vi "_MainOpenMV_New.vi"() -> ()   [LabVIEW 2017]
panel:
  in  "clear":bool
  in  "Set Threshold":bool
  out "Plots":T1
  out "Lab":string="[10,90,-40,40,-40,40]"
  out "Tx Buffer":string
  in  "Play":bool
  in  "Serial Port":refnum<visa-resource-name>="ASRL30::INSTR"
  out "Version":string
  in  "Connect":bool
  out "FPS":dbl format="%#.2g"
  in  "Tabs":enum32{"Simple View", "REPL", "Python"}(tab)
  in  "WiFi":cluster{"SSID":string, "Key":string}
  in  "SystemLink":T2={"APIKey"="", "Tag"="", "Type"="STRING"}
  in  "Destination":T3(ring)
  out "Value":dbl(graph)
  in  "ROI":T4={"left"=0, "top"=0, "right"=320, "bottom"=240}
  in  "Set ROI":bool
  in  "View":T5(ring)
  in  "Ctrl D":bool
  in  "Grab Script":bool
  in  "Line":u8(slide) scale=0.0..27.0
  in  "Send Line":bool
  out "Console":string
  in  "Notepad":string
  in  "Ctrl C":bool
  out "rows":string="  1\n  2\n  3\n  4\n  5\n  6\n  7\n  8\n  9\n 10\n 11\n 12\n 13\n 14\n 15\n 16\n 17\n 18\n 19\n 20\n 21\n"
  in  "Script":string="# Show Color - lmean\n\nimport sensor, image, time\n\nsensor.reset()\nsensor.set_pixformat(sensor.RGB565)\nsensor.set_framesize(sensor.QVGA)\nsensor.skip_frames(time = 2000)\n\nsensor.set_auto_gain(False)\nsensor.set_auto_whitebal(False) \n\nclock = time.clock()\n\n\n\nwhile(True):\n    clock.tick()\n    img = sensor.snapshot()\n    \n    print(img.statistics()[0])\n"
  in  "New":bool
  in  "Load":bool
  in  "Save":bool
  in  "File":path
  in  "startCode":string="# Hello World Example\n#\n# Welcome to the OpenMV IDE! Click on the green run arrow button below to run the script!\n\nimport sensor, image, time\n\nsensor.reset()                      # Reset and initialize the sensor.\nsensor.set_pixformat(sensor.RGB565) # Set pixel format to RGB565 (or GRAYSCALE)\nsensor.set_framesize(sensor.QVGA)   # Set frame size to QVGA (320x240)\nsensor.skip_frames(time = 2000)     # Wait for settings take effect.\nclock = time.clock()                # Create a clock object to track the FPS.\n\nwhile(True):\n    clock.tick()                    # Update the FPS clock.\n    img = sensor.snapshot()         # Take a picture and return the image.\n    print(clock.fps())              # Note: OpenMV Cam runs about half as fast when connected\n                                    # to the IDE. The FPS should increase once disconnected.\n"
  out "Size":string
  in  "stop":bool
  out "image":picture
  # "LabVIEW OpenMV"
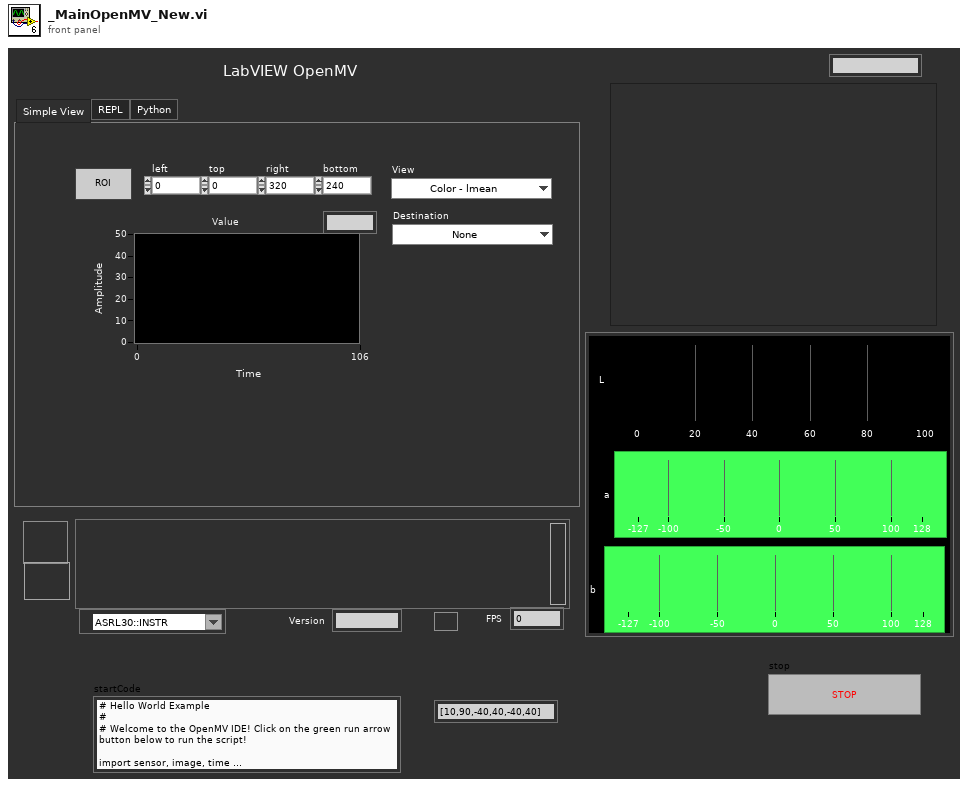
[diagram p1: front panel]
types:
  T1 = cluster{"L":dbl[], "a":cluster{i32, i32, dbl[]}, "b":cluster{i32, i32, dbl[]}}
  T2 = cluster{"APIKey":string, "Tag":string, "Type":string}
  T3 = enum16{"None", "UART (Tx-4, Rx-5)", "SPI (MOSI - 0, MISO-1, SCK-2)", "I2C (SCL-4,SDA-5)", "WiFi"}
  T4 = cluster{"left":i32, "top":i32, "right":i32, "bottom":i32}
  T5 = enum16{"Color - lmean", "Color - lmode", "Greyscale - mean", "Greyscale - mode", "Track Blobs", "Track Faces", "QRCode"}
  T6 = enum8{"Enabled", "Disabled", "Disabled and Grayed Out"}
  T7 = enum16{"Color - lmean", "Color - lmode", "Greyscale - mean", "Greyscale - mode", "Track Blobs", "Track Faces", "Optical Flow"}
  T8 = typedef "imagedata.ctl" = cluster{"image type":i32, "image depth":i32, "image":u8[], "mask":u8[], "colors":u32[], "Rectangle":cluster{"left":i16, "top":i16, "right":i16, "bottom":i16}}
  T9 = cluster{"left":i16, "top":i16, "right":i16, "bottom":i16}
  T10 = typedef "eventvkey.ctl" = enum16{"ASCII", "Enter", "Return", "Shift", "Ctrl", "Alt", "Cmd", "Opt", "Caps", "NumLock", "Clear", "Break", "Up", "Down", "Left", "Right", "Insert", "Delete", "Home", "End", "PageUp", "PageDown", "Escape", "Help", "Pause", "ScrollLock", "F1", "F2", "F3", "F4", "F5", "F6", "F7", "F8", "F9", "F10", "F11", "F12", "F13", "F14", "F15", "F16", "F17", "F18", "F19", "F20", "F21", "F22", "F23", "F24", "Play", "VolumeUp", "VolumeDown", "Mute", "Two Byte Char"}
  T11 = cluster{"Shift":bool, "Ctrl":bool, "Alt":bool, "Cmd":bool, "Opt":bool}
  T12 = cluster{"Char":i16, "VKey":T10, "ScanCode":i16, "Mods":cluster{"Num Pad":bool, "Menu Key":bool}, "PlatMods":cluster{"Shift":bool, "Ctrl":bool, "Alt":bool, "Cmd":bool, "Opt":bool}, "FocusObj":refnum<vi>}
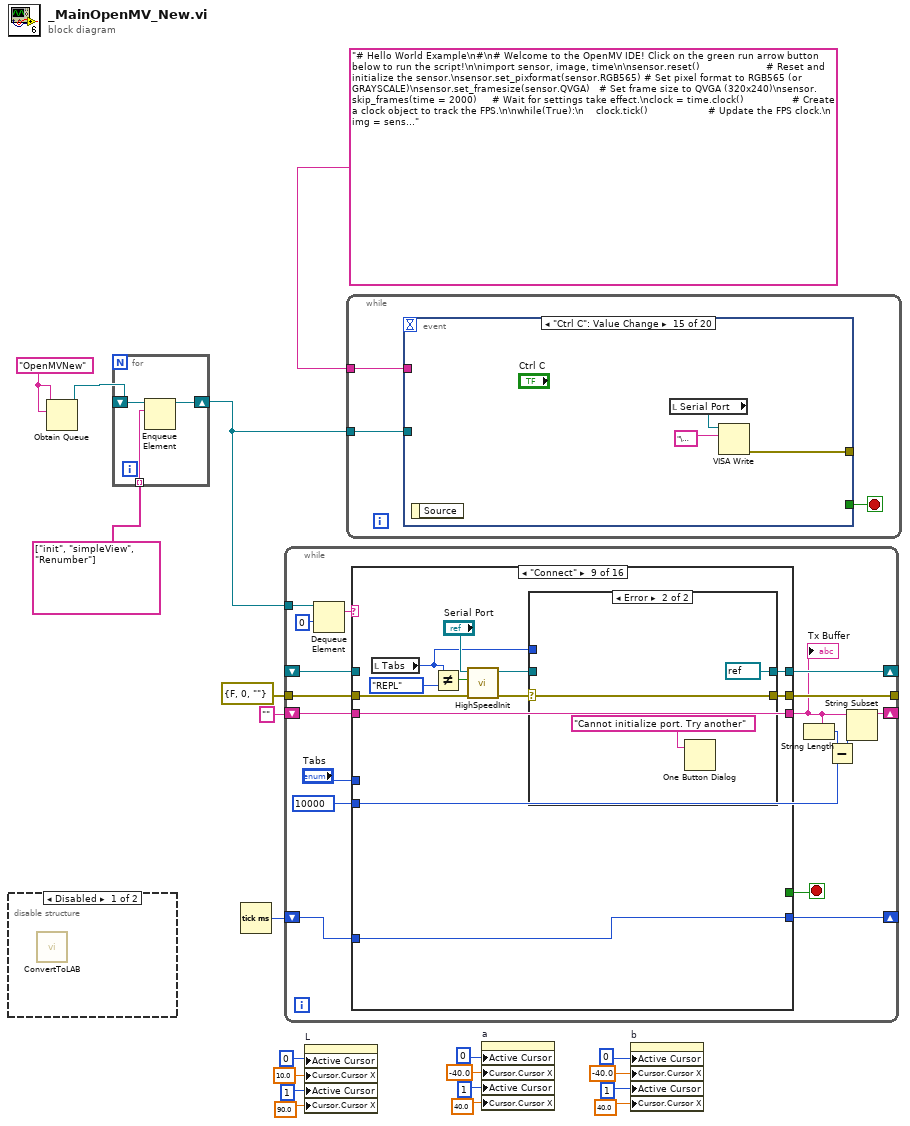
[diagram p0: block diagram]
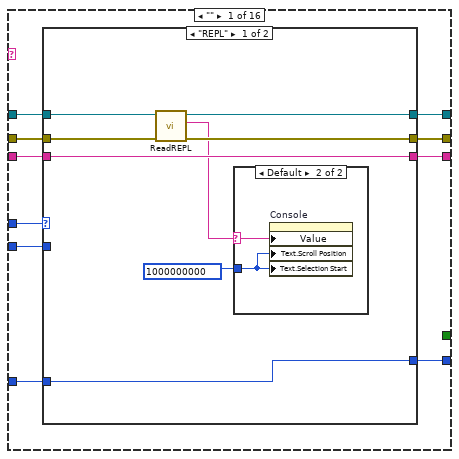
[diagram p3: hidden frame]
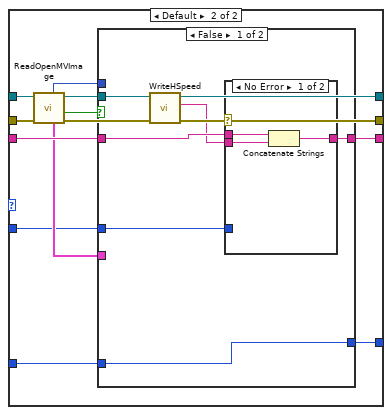
[diagram p5: hidden frame]
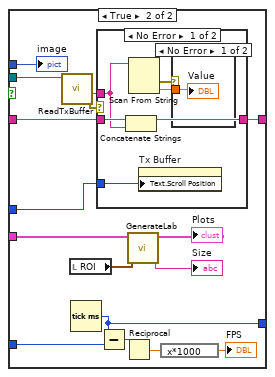
[diagram p7: hidden frame]
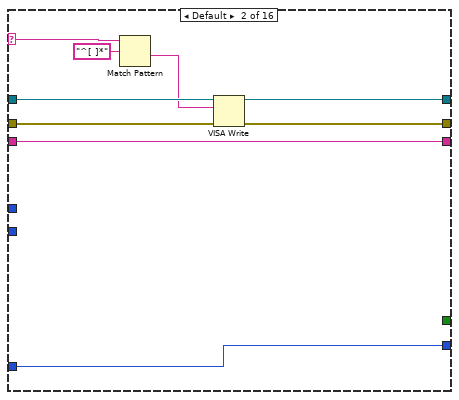
[diagram p10: hidden frame]
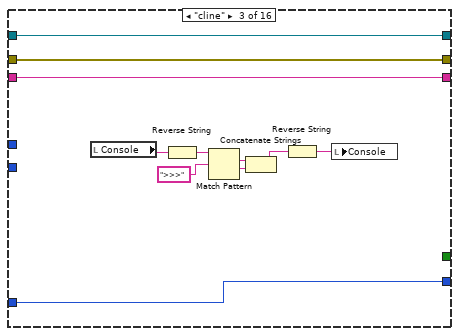
[diagram p11: hidden frame]
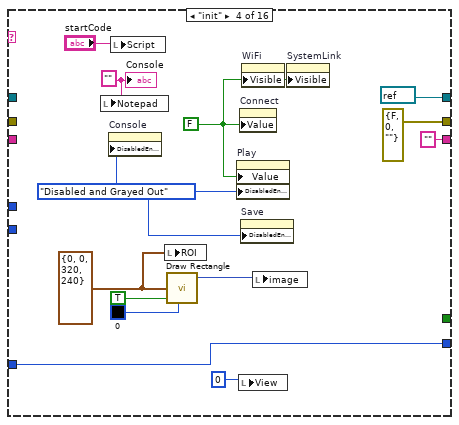
[diagram p12: hidden frame]
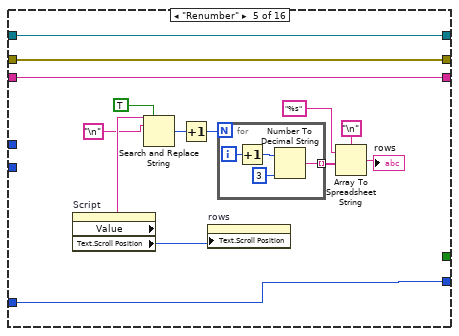
[diagram p13: hidden frame]
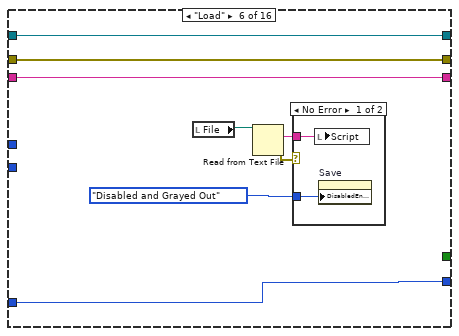
[diagram p14: hidden frame]
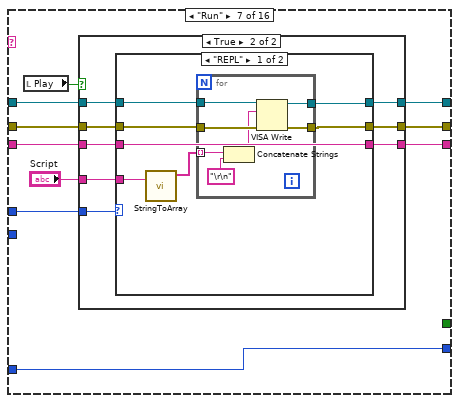
[diagram p16: hidden frame]
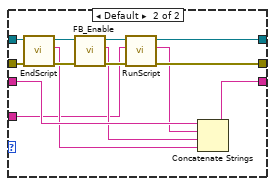
[diagram p18: hidden frame]
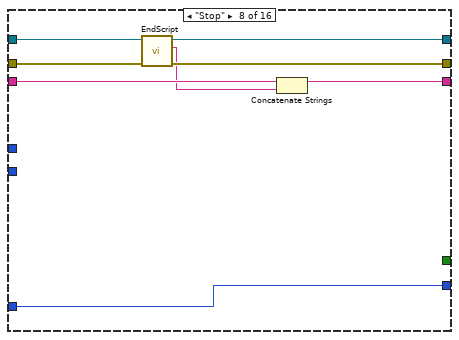
[diagram p19: hidden frame]
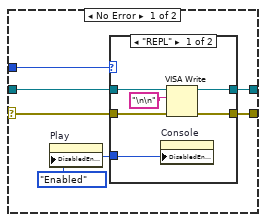
[diagram p20: hidden frame]
diagram:
  w20 = "OpenMVNew" ("name (unnamed)")
  n1 = disable-structure shown="Disabled" {
    frame Disabled {
      n2 = call <userlib>:"ConvertToLAB.vi"() -> ()  [unwired: 9 in, 3 out]
    }
    frame Enabled {
    }
  }
  n3 = Obtain Queue(name (unnamed)=w20, element data type=w20) -> (queue out=w15:refnum<queue>)  [unwired: 3 in, 2 out]
  n4 = for {
    shift-right: [w23] -> w17
    shift-left: w15 -> [w22]
    tunnel: string[] ["init", "simpleView", "Renumber"] -> [w21] mode=indexing
    n5 = Enqueue Element(queue=w22, element=w21) -> (queue out=w23:refnum<queue>)  [unwired: 2 in, 2 out]
  }
  n6 = Tick Count (ms)() -> (millisecond timer value=w18:u32)
  n7 = while {
    tunnel: w17 -> [w39]
    shift-right: [w36] -> _
    shift-left: _ -> [w37]
    shift-right: [w30] -> _
    shift-left: "" ("Tx Buffer") -> [w29]
    tunnel: errorcluster {"status"=FALSE, "code"=0, "source"=""} ("error out") -> [w34]
    tunnel: [w33] -> _
    shift-right: [w32] -> _
    shift-left: w18 -> [w31]
    stop <- w35 stop-if-true
    w27 = 10000 ("length (rest)")
    n8 = Dequeue Element(queue=w39, timeout in ms (-1)=0) -> (element=w38:string)  [unwired: 1 in, 3 out]
    n9 = case shown="\"Connect\"" w38 {
      selector: w38 -> [_ w110 _ _ _ _ _ _ _ _ _ _ _ _ _ _]
      tunnel: w37 -> [w50 w114 w125 _ w154 w166 w178 w225 _ w264 w279 w303 w311 w334 w341 w347]
      tunnel: [w47 w111 w125 refnum<visa-resource-name> refnum ("VISA Refnum out") w154 w166 w176 w222 w235 refnum<visa-resource-name> refnum ("VISA Refnum out") w279 w303 w311 w334 w341 w347] -> w36
      tunnel: [w48 w112 w124 errorcluster {"status"=FALSE, "code"=0, "source"=""} ("error out") w153 w165 w175 w223 w234 w262 w278 w302 w310 w333 w340 w346] -> w33
      tunnel: w34 -> [w49 w113 w124 _ w153 w165 w177 w224 w233 w263 w278 w302 w310 w333 w340 w346]
      tunnel: w29 -> [w46 w116 w127 _ w152 w164 w174 w219 w232 w266 w277 w301 w309 w336 _ w345]
      tunnel: [w45 w116 w127 "" ("Tx Buffer") w152 w164 w173 w220 w232 w266 w277 w301 w309 w336 "" ("Tx Buffer") w345] -> w26
      tunnel: [_ _ _ _ _ _ _ _ _ _ _ _ _ _ _ TRUE] -> w35
      tunnel: [w44 w115 w126 w137 w151 w163 w172 w221 w230 w260 w274 w300 w308 w335 w342 w343] -> w32
      tunnel: w31 -> [w43 w115 w126 w137 w151 w163 w172 w221 w230 w260 w274 w300 w308 w335 w342 w343]
      tunnel: w27 -> [w42 _ _ _ _ _ _ _ _ _ _ _ _ _ _ _]
      tunnel: "Tabs" -> [w41 _ _ _ _ _ w170 _ _ _ _ _ _ _ _ _]
      frame "" {
        n10 = case shown="\"REPL\"" w41 {
          tunnel: w50 -> [w58 w70]
          tunnel: w49 -> [w57 w69]
          tunnel: [w55 w68] -> w48
          tunnel: [w56 w67] -> w47
          tunnel: w46 -> [w54 w66]
          tunnel: [w54 w65] -> w45
          tunnel: [w53 w64] -> w44
          tunnel: w43 -> [w53 w63]
          tunnel: w42 -> [_ w61]
          frame "REPL" {
            n11 = call <userlib>:"ReadREPL.vi"("error in (no error)"=w57, "VISA Refnum in"=w58) -> ("error out"=w55:errorcluster, "String"=w51:string, "VISA Refnum out"=w56:refnum<visa-resource-name>)  [unwired: 7 in]
            n12 = case shown="Default" w51 {
              selector: w51 -> [_ w59]
              tunnel: u32 1000000000 ("Text.Selection:Start") -> [_ w60]
              frame "" {
              }
              frame Default {
                n13 = property on="Console" class="Str"("Value"=w59, "Text.Scroll Position"=w60, "Text.Selection Start"=w60) -> ()  [unwired: 2 in, 2 out]
              }
            }
          }
          frame Default {
            n14 = call <userlib>:"ReadOpenMVImage.vi"("error in"=w69, "VISA Refnum in"=w70) -> ("error out"=w68:errorcluster, "Good?"=w72:bool, "VISA Refnum out"=w67:refnum<visa-resource-name>, "image data"=w62:T8, "new picture"=w71:picture)  [unwired: 4 in, 1 out]
            n15 = case shown="False" w72 {
              tunnel: w71 -> [_ w93]
              tunnel: w67 -> [w75 w99]
              tunnel: [w77 w89] -> w65
              tunnel: w66 -> [w78 w87]
              tunnel: [w79 w98] -> w64
              tunnel: w63 -> [w79 w97]
              tunnel: w62 -> [_ w91]
              tunnel: w61 -> [w76 w84]
              frame False {
                n16 = call <userlib>:"WriteHSpeed.vi"("VISA Refnum in"=w75) -> ("error out"=w73:errorcluster, "read buffer"=w74:string)  [unwired: 8 in, 1 out]
                n17 = case shown="No Error" w73 {
                  tunnel: w74 -> [w82 _]
                  tunnel: w78 -> [w81 w83]
                  tunnel: [w80 w83] -> w77
                  tunnel: w76 -> [_ _]
                  frame No Error {
                    n18 = Concatenate Strings(w81, w82) -> (w80:string)
                  }
                  frame Error {
                  }
                }
              }
              frame True {
                n19 = call <userlib>:"ReadTxBuffer.vi"("VISA Refnum in"=w99) -> ("error out"=w85:errorcluster, "Tx Buffer"=w86:string)  [unwired: 7 in, 2 out]
                n20 = local read "ROI"() -> (w90:T4)
                n21 = Tick Count (ms)() -> (millisecond timer value=w98:u32)
                n22 = case shown="No Error" w85 {
                  tunnel: [w105 w107] -> w89
                  tunnel: w87 -> [w102 w107]
                  tunnel: w86 -> [w101 _]
                  tunnel: w84 -> [w100 _]
                  frame No Error {
                    n23 = Concatenate Strings(w102, w101) -> (w105:string)
                    n24 = Scan From String(input string=w101) -> (error out=w104:errorcluster, output 1=w103:dbl)  [unwired: 4 in, 2 out]
                    n25 = property on="Tx Buffer" class="Str"("Text.Scroll Position"=w100) -> ()  [unwired: 2 in, 2 out]
                    n26 = case shown="No Error" w104 {
                      tunnel: w103 -> [w106 _]
                      frame No Error {
                        "Value" <- w106
                      }
                      frame Error {
                      }
                    }
                  }
                  frame Error {
                  }
                }
                n27 = Subtract(x=w98, y=w97) -> (x-y=w94:u32)
                n28 = Reciprocal(x=w94) -> (1/x=w96:dbl)
                n29 = call <userlib>:"GenerateLab.vi"("ROI"=w90, "image data"=w91) -> ("Dimensions"=→"Size":string, "Plots"=→"Plots":T1)  [unwired: 8 in]
                n30 = expression code="x*1000"(w96) -> (→"FPS":dbl)
                "image" <- w93
              }
            }
          }
        }
      }
      frame Default {
        n31 = Match Pattern(string=w110, regular expression="^[ ]*") -> (after substring=w109:string)  [unwired: 1 in, 3 out]
        n32 = VISA Write(VISA resource name=w114, write buffer=w109, error in (no error)=w113) -> (VISA resource name out=w111:refnum<visa-resource-name>, error out=w112:errorcluster)  [unwired: 1 out]
      }
      frame "cline" {
        n33 = local read "Console"() -> (w117:string)
        n34 = Reverse String(1:w117) -> (0:w123:string)
        n35 = Match Pattern(string=w123, regular expression=">>>") -> (match substring=w120:string, after substring=w121:string)  [unwired: 1 in, 2 out]
        n36 = Concatenate Strings(w120, w121) -> (w119:string)
        n37 = Reverse String(1:w119) -> (0:w118:string)
        n38 = local write "Console"(w118) -> ()
      }
      frame "init" {
        w130 = "" ("Tx Buffer")
        w132 = T9 {"left"=0, "top"=0, "right"=320, "bottom"=240} ("rect")
        w129 = T6."Disabled and Grayed Out" ("Disabled")
        w131 = FALSE ("Connect")
        n39 = local write "Notepad"(w130) -> ()
        n40 = property on="Console" class="Str"("DisabledEnum"=w129) -> ()  [unwired: 2 in, 2 out]
        n41 = local write "Script"("startCode") -> ()
        n42 = local write "ROI"(w132) -> ()
        n43 = call <vilib>:"Draw Rectangle.vi"("rect"=w132, "fill?(F)"=TRUE, "color(black)"=u32 0) -> ("new picture"=w134:picture)  [unwired: 6 in]
        n44 = property on="Play" class="Bool (strict)"("Value"=w131, "DisabledEnum"=w129) -> ()  [unwired: 2 in, 2 out]
        n45 = local write "View"(i16 0 ("left")) -> ()
        n46 = property on="Connect" class="Bool (strict)"("Value"=w131) -> ()  [unwired: 2 in, 2 out]
        n47 = property on="Save" class="Bool"("DisabledEnum"=w129) -> ()  [unwired: 2 in, 2 out]
        n48 = property on="WiFi" class="Clust (strict)"("Visible"=w131) -> ()  [unwired: 2 in, 2 out]
        n49 = local write "image"(w134) -> ()
        n50 = property on="SystemLink" class="Clust (strict)"("Visible"=w131) -> ()  [unwired: 2 in, 2 out]
        "Console" <- w130
      }
      frame "Renumber" {
        n51 = property on="Script" class="Str"() -> ("Value"=w150:string, "Text.Scroll Position"=w149:u32)  [unwired: 2 in, 2 out]
        n52 = Search and Replace String(replace all?=TRUE ("replace all? (F)"), input string=w150, search string="\n") -> (number of replacements=w148:i32)  [unwired: 5 in, 3 out]
        n53 = Increment(x=w148) -> (x+1=w141:i32)
        n54 = property on="rows" class="Str"("Text.Scroll Position"=w149) -> ()  [unwired: 2 in, 2 out]
        n55 = for {
          N: w141 -> [_]
          tunnel: [w158] -> w146 mode=indexing
          i -> [w155]
          n56 = Increment(x=w155) -> (x+1=w157:i32)
          n57 = Number To Decimal String(number=w157, width (-)=i16 3) -> (decimal integer string=w158:string)
        }
        n58 = Array To Spreadsheet String(delimiter (Tab)="\n", array=w146, 3:"%s" ("format string")) -> (spreadsheet string=→"rows":string)
      }
      frame "Load" {
        n59 = local read "File"() -> (w162:path)
        n60 = Read from Text File(file (use dialog)=w162) -> (text=w159:string, error out=w160:errorcluster)  [unwired: 3 in, 2 out]
        n61 = case shown="No Error" w160 {
          tunnel: T6."Disabled and Grayed Out" ("Disabled") -> [w168 _]
          tunnel: w159 -> [w167 _]
          frame No Error {
            n62 = local write "Script"(w167) -> ()
            n63 = property on="Save" class="Bool"("DisabledEnum"=w168) -> ()  [unwired: 2 in, 2 out]
          }
          frame Error {
          }
        }
      }
      frame "Run" {
        n64 = local read "Play"() -> (w171:bool)
        n65 = case shown="True" w171 {
          tunnel: w178 -> [w181 w189]
          tunnel: w177 -> [w180 w188]
          tunnel: [w181 w187] -> w176
          tunnel: [w180 w186] -> w175
          tunnel: w174 -> [w179 w184]
          tunnel: [w179 w185] -> w173
          tunnel: w170 -> [_ w183]
          tunnel: "Script" -> [_ w182]
          frame False {
          }
          frame True {
            n66 = case shown="\"REPL\"" w183 {
              tunnel: w189 -> [w195 w213]
              tunnel: w188 -> [w194 w212]
              tunnel: [w192 w211] -> w187
              tunnel: [w193 w210] -> w186
              tunnel: [w190 w209] -> w185
              tunnel: w184 -> [w190 w208]
              tunnel: w182 -> [w191 w204]
              frame "REPL" {
                n67 = call <userlib>:"StringToArray.vi"("write buffer"=w191) -> ("Array"=w196:string[])  [unwired: 10 in]
                n68 = for {
                  tunnel: w196 -> [w198] mode=indexing
                  tunnel: w195 -> [w203]
                  tunnel: w194 -> [w202]
                  tunnel: [w201] -> w193
                  tunnel: [w200] -> w192
                  n69 = Concatenate Strings(w198, "\r\n" ("write buffer")) -> (w197:string)
                  n70 = VISA Write(VISA resource name=w203, write buffer=w197, error in (no error)=w202) -> (VISA resource name out=w200:refnum<visa-resource-name>, error out=w201:errorcluster)  [unwired: 1 out]
                }
              }
              frame Default {
                n71 = call <userlib>:"EndScript.vi"("error in (no error)"=w212, "VISA Refnum in"=w213) -> ("error out"=w217:errorcluster, "Tx for stopping code"=w205:string, "VISA Refnum out"=w216:refnum<visa-resource-name>)  [unwired: 7 in]
                n72 = call <userlib>:"FB_Enable.vi"("error in"=w217, "VISA Refnum in"=w216) -> ("error out"=w215:errorcluster, "Reply"=w206:string, "VISA Refnum out"=w214:refnum<visa-resource-name>)  [unwired: 7 in]
                n73 = call <userlib>:"RunScript.vi"("error in"=w215, "script"=w204, "VISA Refnum in"=w214) -> ("error out"=w210:errorcluster, "Tx"=w207:string, "VISA Refnum out"=w211:refnum<visa-resource-name>)  [unwired: 6 in]
                n74 = Concatenate Strings(w208, w207, w206, w205) -> (w209:string)
              }
            }
          }
        }
      }
      frame "Stop" {
        n75 = call <userlib>:"EndScript.vi"("error in (no error)"=w224, "VISA Refnum in"=w225) -> ("error out"=w223:errorcluster, "Tx for stopping code"=w218:string, "VISA Refnum out"=w222:refnum<visa-resource-name>)  [unwired: 7 in]
        n76 = Concatenate Strings(w219, w218) -> (w220:string)
      }
      frame "Connect" {
        n77 = local read "Tabs"() -> (w227:enum32{"Simple View", "REPL", "Python"})
        n78 = Not Equal?(x=w227, y=enum32{"Simple View", "REPL", "Python"}."REPL") -> (x != y?=w229:bool)
        n79 = call <userlib>:"HighSpeedInit.vi"("error in"=w233, "Fast"=w229, "VISA Refnum in"="Serial Port") -> ("error out"=w226:errorcluster, "VISA Refnum out"=w236:refnum<visa-resource-name>)  [unwired: 7 in]
        n80 = case shown="Error" w226 {
          selector: w226 -> [w237 w255]
          tunnel: w236 -> [w242 _]
          tunnel: [w241 refnum<visa-resource-name> refnum ("VISA Refnum out")] -> w235
          tunnel: [w240 w255] -> w234
          tunnel: w227 -> [w239 _]
          frame No Error {
            w238 = T6."Enabled" ("Disabled")
            n81 = property on="Play" class="Bool (strict)"("DisabledEnum"=w238) -> ()  [unwired: 2 in, 2 out]
            n82 = case shown="\"REPL\"" w239 {
              tunnel: w237 -> [w246 w253]
              tunnel: w242 -> [w248 w252]
              tunnel: [w244 w250] -> w241
              tunnel: [w245 w249] -> w240
              tunnel: w238 -> [w243 _]
              frame "REPL" {
                n83 = property on="Console" class="Str"("DisabledEnum"=w243) -> ()  [unwired: 2 in, 2 out]
                n84 = VISA Write(VISA resource name=w248, write buffer="\n\n", error in (no error)=w246) -> (VISA resource name out=w244:refnum<visa-resource-name>, error out=w245:errorcluster)  [unwired: 1 out]
              }
              frame Default {
                n85 = call <userlib>:"AskVersion.vi"("error in"=w253, "VISA Refnum in"=w252) -> ("error out"=w249:errorcluster, "Version"=→"Version":string, "VISA Refnum out"=w250:refnum<visa-resource-name>)  [unwired: 7 in]
              }
            }
          }
          frame Error {
            n86 = One Button Dialog(message="Cannot initialize port. Try another") -> ()  [unwired: 1 in, 1 out]
          }
        }
      }
      frame "Disconnect" {
        w257 = T6."Disabled and Grayed Out" ("Disabled")
        n87 = local read "Tabs"() -> (w258:enum32{"Simple View", "REPL", "Python"})
        n88 = case shown="\"REPL\"" w258 {
          tunnel: [w269 w273] -> w265
          tunnel: w264 -> [w269 w272]
          tunnel: w263 -> [w268 w271]
          tunnel: [w268 w270] -> w262
          frame "REPL" {
          }
          frame Default {
            n89 = call <userlib>:"EndScript.vi"("error in (no error)"=w271, "VISA Refnum in"=w272) -> ("error out"=w270:errorcluster, "VISA Refnum out"=w273:refnum<visa-resource-name>)  [unwired: 7 in, 1 out]
          }
        }
        n90 = call <userlib>:"CloseHS.vi"("error in (no error)"=w262, "VISA Refnum in"=w265) -> ()  [unwired: 10 in]
        n91 = local write "Connect"(FALSE ("Connect")) -> ()
        n92 = property on="Play" class="Bool (strict)"("Value"=FALSE ("Play"), "DisabledEnum"=w257) -> ()  [unwired: 2 in, 2 out]
        n93 = property on="Console" class="Str"("DisabledEnum"=w257) -> ()  [unwired: 2 in, 2 out]
      }
      frame "ROI" {
        n94 = local read "image"() -> (w275:picture)
        n95 = call <userlib>:"OpenMV_SelectROI.vi"("image"=w275) -> ("Rect"=w276:T4)  [unwired: 2 in]
        n96 = local write "ROI"(w276) -> ()
      }
      frame "Lab" {
        n97 = property on="L" class="WFGraph (strict)"("Active Cursor"=u32 0, "Active Cursor"=u32 1) -> ("Cursor.Cursor X"=w293:dbl, "Cursor.Cursor X"=w292:dbl)  [unwired: 2 in, 2 out]
        n98 = property on="a" class="WFGraph (strict)"("Active Cursor"=u32 0, "Active Cursor"=u32 1) -> ("Cursor.Cursor X"=w294:dbl, "Cursor.Cursor X"=w295:dbl)  [unwired: 2 in, 2 out]
        n99 = property on="b" class="WFGraph (strict)"("Active Cursor"=u32 0, "Active Cursor"=u32 1) -> ("Cursor.Cursor X"=w296:dbl, "Cursor.Cursor X"=w297:dbl)  [unwired: 2 in, 2 out]
        n100 = Max & Min(x=w293, y=w292) -> (max(x,y)=w285:dbl, min(x,y)=w284:dbl)
        n101 = Max & Min(x=w294, y=w295) -> (max(x,y)=w283:dbl, min(x,y)=w282:dbl)
        n102 = Max & Min(x=w296, y=w297) -> (max(x,y)=w280:dbl, min(x,y)=w281:dbl)
        n103 = Format Into String(format string="[%d,%d,%d,%d,%d,%d]", w284, w285, w282, w283, w281, w280) -> (resulting string=→"Lab":string)  [unwired: 2 in, 1 out]
      }
      frame "LabPopup" {
        n104 = local read "image"() -> (w306:picture)
        n105 = local read "ROI"() -> (w304:T4)
        n106 = call <userlib>:"OpenMV_SelectLab.vi"("ROI"=w304, "image"=w306) -> ("ROI out"=w305:T4, "thresholds"=w307:dbl[])
        n107 = for {
          tunnel: w307 -> [w312] mode=indexing
          i -> [w316]
          n108 = Quotient & Remainder(x=w316, y=2) -> (x-y*floor(x/y)=w313:i32, floor(x/y)=w314:i32)
          n109 = case shown="0" w314 {
            tunnel: w313 -> [_ w318 w320 w322]
            tunnel: w312 -> [_ w317 w319 w321]
            frame Default {
            }
            frame 0 {
              n110 = property on="L" class="WFGraph (strict)"("Active Cursor"=w318, "Cursor.Cursor X"=w317) -> ()  [unwired: 2 in, 2 out]
            }
            frame 1 {
              n111 = property on="a" class="WFGraph (strict)"("Active Cursor"=w320, "Cursor.Cursor X"=w319) -> ()  [unwired: 2 in, 2 out]
            }
            frame 2 {
              n112 = property on="b" class="WFGraph (strict)"("Active Cursor"=w322, "Cursor.Cursor X"=w321) -> ()  [unwired: 2 in, 2 out]
            }
          }
        }
        n113 = local write "ROI"(w305) -> ()
      }
      frame "simpleView" {
        n114 = Equal?(x=T7."Track Blobs", y="View") -> (x = y?=w329:bool)
        n115 = local read "Lab"() -> (w326:string)
        n116 = for {
          N: 2 -> [_]
          tunnel: w329 -> [w338]
          i -> [w337]
          n117 = property on="L" class="WFGraph (strict)"("Active Cursor"=w337, "Cursor.Visible"=w338) -> ()  [unwired: 2 in, 2 out]
          n118 = property on="a" class="WFGraph (strict)"("Active Cursor"=w337, "Cursor.Visible"=w338) -> ()  [unwired: 2 in, 2 out]
          n119 = property on="b" class="WFGraph (strict)"("Active Cursor"=w337, "Cursor.Visible"=w338) -> ()  [unwired: 2 in, 2 out]
        }
        n120 = call <userlib>:"SensorOperation.vi"("SystemLink"="SystemLink", "WiFi"="WiFi", "ROI"="ROI", "Lab"=w326, "Destination"="Destination", "View"="View") -> ("startCode"=w332:string)  [unwired: 5 in]
        n121 = local write "Script"(w332) -> ()
      }
      frame "Clear" {
      }
      frame "Done" {
      }
    }
    "Tx Buffer" <- w26
    n122 = String Length(string=w26) -> (length=w28:i32)
    n123 = Subtract(x=w28, y=w27) -> (x-y=w25:i32)
    n124 = String Subset(string=w26, offset (0)=w25) -> (substring=w30:string)  [unwired: 1 in]
  }
  n125 = property on="L" class="WFGraph (strict)"("Active Cursor"=u32 0, "Cursor.Cursor X"=10.0 ("Cursor.Cursor Position:Cursor X"), "Active Cursor"=u32 1, "Cursor.Cursor X"=90.0 ("Cursor.Cursor Position:Cursor X")) -> ()  [unwired: 2 in, 2 out]
  n126 = while {
    tunnel: w17 -> [w349]
    tunnel: "# Hello World Example\n#\n# Welcome to the OpenMV IDE! Click on the green run arrow button below to run the script!\n\nimport sensor, image, time\n\nsensor.reset()                      # Reset and initialize the sensor.\nsensor.set_pixformat(sensor.RGB565) # Set pixel format to RGB565 (or GRAYSCALE)\nsensor.set_framesize(sensor.QVGA)   # Set frame size to QVGA (320x240)\nsensor.skip_frames(time = 2000)     # Wait for settings take effect.\nclock = time.clock()                # Create a clock object to track the FPS.\n\nwhile(True):\n    clock.tick()                    # Update the FPS clock.\n    img = sensor.snapshot()         # Take a picture and return the image.\n    print(clock.fps())              # Note: OpenMV Cam runs about half as fast when connected\n                                    # to the IDE. The FPS should increase once disconnected.\n" ("startCode") -> [w348]
    stop <- w350 stop-if-true
    n127 = event shown="[14] \"Ctrl C\": Value Change" {
      selector: _ -> [_ _ _ _ _ _ _ _ _ _ _ _ _ _ _ _ _ _ _ _]
      dyn-events: _ -> [_ _ _ _ _ _ _ _ _ _ _ _ _ _ _ _ _ _ _ _]
      timeout: _ -> [_ _ _ _ _ _ _ _ _ _ _ _ _ _ _ _ _ _ _ _]
      tunnel: [_ "stop" _ _ _ _ _ _ _ _ _ _ _ _ _ _ _ _ _ _] -> w350
      tunnel: w349 -> [_ w353 w363 w372 w377 w379 _ w387 _ w415 w421 w427 w435 w437 _ _ _ w456 _ w464]
      tunnel: w348 -> [_ _ _ _ _ _ w383 _ _ _ _ _ _ _ _ _ _ _ _ _]
      tunnel: [_ _ _ _ _ _ _ _ _ _ _ _ _ _ w439 w442 _ _ _ _] -> _
      event Timeout {
        n128 = event-data() -> ()  [unwired: 1 in, 1 out]
      }
      event "stop": Value Change {
        n129 = event-data() -> ()  [unwired: 1 in, 1 out]
        n130 = local read "Connect"() -> (w351:bool)
        n131 = case shown="True" w351 {
          tunnel: w353 -> [w356 w359]
          tunnel: [w356 w358] -> w352
          frame False {
          }
          frame True {
            n132 = Enqueue Element(queue=w359, element="Disconnect") -> (queue out=w358:refnum<queue>)  [unwired: 2 in, 2 out]
          }
        }
        n133 = Enqueue Element(queue=w352, element="Done") -> ()  [unwired: 2 in, 3 out]
      }
      event "Tabs": Value Change {
        n134 = event-data() -> ()  [unwired: 1 in, 1 out]
        n135 = local read "Tabs"() -> (w360:enum32{"Simple View", "REPL", "Python"})
        n136 = case shown="\"REPL\"" w360 {
          tunnel: w363 -> [w364 w367]
          tunnel: [w364 w365] -> w362
          frame Default {
          }
          frame "REPL" {
            n137 = Enqueue Element(queue=w367, element="Disconnect") -> (queue out=w365:refnum<queue>)  [unwired: 2 in, 2 out]
          }
        }
        n138 = Enqueue Element(queue=w362, element="Renumber") -> ()  [unwired: 2 in, 3 out]
      }
      event "Play": Value Change {
        n139 = event-data() -> ()  [unwired: 1 in, 1 out]
        n140 = Select(t="Run" ("element"), s="Play", f="Stop" ("element")) -> (s? t:f=w368:string)
        n141 = Enqueue Element(queue=w372, element=w368) -> ()  [unwired: 2 in, 3 out]
      }
      event "Connect": Value Change {
        n142 = event-data() -> ()  [unwired: 1 in, 1 out]
        n143 = Select(t="Connect" ("element"), s="Connect", f="Disconnect" ("element")) -> (s? t:f=w375:string)
        n144 = Enqueue Element(queue=w377, element=w375) -> ()  [unwired: 2 in, 3 out]
      }
      event "Script": Value Change; "Script": Mouse Up {
        n145 = event-data() -> ()  [unwired: 1 in, 1 out]
        n146 = Enqueue Element(queue=w379, element="Renumber") -> ()  [unwired: 2 in, 3 out]
        n147 = property on="Save" class="Bool"("DisabledEnum"=T6."Enabled" ("Disabled")) -> ()  [unwired: 2 in, 2 out]
      }
      event "New": Value Change {
        n148 = event-data() -> ()  [unwired: 1 in, 1 out]
        n149 = property on="Save" class="Bool"() -> ("DisabledEnum"=w382:T6)  [unwired: 2 in, 2 out]
        n150 = call <userlib>:"CheckReplace.vi"("DisabledEnum"=w382) -> ("Replace?"=w381:bool)  [unwired: 10 in]
        n151 = case shown="True" w381 {
          tunnel: w383 -> [_ w385]
          frame False {
          }
          frame True {
            n152 = local write "Script"(w385) -> ()
            n153 = property on="Save" class="Bool"("DisabledEnum"=T6."Enabled" ("Disabled")) -> ()  [unwired: 2 in, 2 out]
            n154 = local write "File"(path "" ("File")) -> ()
          }
        }
      }
      event "Load", "File": Value Change {
        n155 = event-data() -> ()  [unwired: 1 in, 1 out]
        n156 = property on="Save" class="Bool"() -> ("DisabledEnum"=w389:T6)  [unwired: 2 in, 2 out]
        n157 = call <userlib>:"CheckReplace.vi"("DisabledEnum"=w389) -> ("Replace?"=w388:bool)  [unwired: 10 in]
        n158 = case shown="True" w388 {
          tunnel: w387 -> [_ w392]
          frame False {
          }
          frame True {
            n159 = call "File Dialog2"() -> ("selected path"=w390:path, "cancelled"=w391:bool)  [unwired: 12 in, 2 out]
            n160 = case shown="False" w391 {
              tunnel: w392 -> [w394 _]
              tunnel: w390 -> [w393 _]
              frame False {
                n161 = local write "File"(w393) -> ()
                n162 = Enqueue Element(queue=w394, element="Load") -> (queue out=w395:refnum<queue>)  [unwired: 2 in, 2 out]
                n163 = Enqueue Element(queue=w395, element="Renumber") -> ()  [unwired: 2 in, 3 out]
              }
              frame True {
              }
            }
          }
        }
      }
      event "Save": Value Change {
        n164 = event-data() -> ()  [unwired: 1 in, 1 out]
        n165 = Empty String/Path?(string/path="File") -> (empty?=w400:bool)
        n166 = case shown="True" w400 {
          tunnel: [w404 w406] -> w403
          tunnel: "File" -> [w404 _]
          tunnel: [_ w405] -> w398
          frame False {
          }
          frame True {
            n167 = call "File Dialog"() -> ("selected path"=w406:path, "cancelled"=w405:bool)  [unwired: 12 in, 2 out]
          }
        }
        n168 = local read "Script"() -> (w402:string)
        n169 = case shown="False" w398 {
          tunnel: w403 -> [w409 _]
          tunnel: w402 -> [w408 _]
          tunnel: T6."Disabled and Grayed Out" ("Disabled") -> [w407 _]
          frame False {
            n170 = Write to Text File(file (use dialog)=w409, text=w408) -> ()  [unwired: 2 in, 3 out]
            n171 = property on="Save" class="Bool"("DisabledEnum"=w407) -> ()  [unwired: 2 in, 2 out]
          }
          frame True {
          }
        }
      }
      event "View", "Destination": Value Change {
        n172 = event-data() -> ()  [unwired: 1 in, 1 out]
        n173 = local read "Destination"() -> (w412:T3)
        n174 = Enqueue Element(queue=w415, element="simpleView") -> (queue out=w413:refnum<queue>)  [unwired: 2 in, 2 out]
        n175 = Enqueue Element(queue=w413, element="Run") -> ()  [unwired: 2 in, 3 out]
        n176 = Equal?(x=w412, y=T3."WiFi") -> (x = y?=w410:bool)
        n177 = property on="WiFi" class="Clust (strict)"("Visible"=w410) -> ()  [unwired: 2 in, 2 out]
        n178 = property on="SystemLink" class="Clust (strict)"("Visible"=w410) -> ()  [unwired: 2 in, 2 out]
      }
      event "Set ROI": Value Change {
        n179 = event-data() -> ()  [unwired: 1 in, 1 out]
        n180 = Enqueue Element(queue=w421, element="ROI") -> (queue out=w420:refnum<queue>)  [unwired: 2 in, 2 out]
        n181 = Enqueue Element(queue=w420, element="simpleView") -> (queue out=w417:refnum<queue>)  [unwired: 2 in, 2 out]
        n182 = Enqueue Element(queue=w417, element="Run") -> ()  [unwired: 2 in, 3 out]
      }
      event "Plots.L", "Plots.a", "Plots.b": Cursor Move {
        n183 = event-data() -> ()  [unwired: 1 in, 1 out]
        n184 = Enqueue Element(queue=w427, element="Lab") -> (queue out=w426:refnum<queue>)  [unwired: 2 in, 2 out]
        n185 = Enqueue Element(queue=w426, element="simpleView") -> (queue out=w423:refnum<queue>)  [unwired: 2 in, 2 out]
        n186 = Enqueue Element(queue=w423, element="Run") -> ()  [unwired: 2 in, 3 out]
      }
      event "Set Threshold": Value Change {
        n187 = event-data() -> ()  [unwired: 1 in, 1 out]
        n188 = Enqueue Element(queue=w435, element="LabPopup") -> (queue out=w431:refnum<queue>)  [unwired: 2 in, 2 out]
        n189 = Enqueue Element(queue=w431, element="Lab") -> (queue out=w430:refnum<queue>)  [unwired: 2 in, 2 out]
        n190 = Enqueue Element(queue=w430, element="simpleView") -> (queue out=w432:refnum<queue>)  [unwired: 2 in, 2 out]
        n191 = Enqueue Element(queue=w432, element="Run") -> ()  [unwired: 2 in, 3 out]
      }
      event "clear": Value Change {
        n192 = event-data() -> ()  [unwired: 1 in, 1 out]
        n193 = Enqueue Element(queue=w437, element="Clear") -> ()  [unwired: 2 in, 3 out]
      }
      event "Ctrl C": Value Change {
        n194 = event-data() -> ()  [unwired: 1 in, 1 out]
        n195 = local read "Serial Port"() -> (w440:refnum<visa-resource-name>)
        n196 = VISA Write(VISA resource name=w440, write buffer="\u0003") -> (error out=w439:errorcluster)  [unwired: 1 in, 2 out]
      }
      event "Ctrl D": Value Change {
        n197 = event-data() -> ()  [unwired: 1 in, 1 out]
        n198 = local read "Serial Port"() -> (w443:refnum<visa-resource-name>)
        n199 = VISA Write(VISA resource name=w443, write buffer="\u0004") -> (error out=w442:errorcluster)  [unwired: 1 in, 2 out]
      }
      event "Line": Value Change {
        n200 = event-data() -> ()  [unwired: 1 in, 1 out]
        n201 = property on="Notepad" class="Str"() -> ("Text.Text"=w450:string)  [unwired: 2 in, 2 out]
        n202 = call <userlib>:"Select.vi"("Line"="Line", "Text.Text"=w450) -> ("scale"=w447:i32, "Text min"=w445:i32, "Text max"=w446:i32)  [unwired: 7 in]
        n203 = property on="Line" class="Slide (strict)"("Scale.Maximum"=w447) -> ()  [unwired: 2 in, 2 out]
        n204 = property on="Notepad" class="Str"("Key Focus"=TRUE, "Text.Selection End"=w446, "Text.Selection Start"=w445) -> ()  [unwired: 2 in, 2 out]
      }
      event "Send Line": Value Change {
        n205 = event-data() -> ()  [unwired: 1 in, 1 out]
        n206 = local read "Line"() -> (w452:u8)
        n207 = call <userlib>:"StringToArray.vi"("write buffer"="Notepad") -> ("Array"=w457:string[])  [unwired: 10 in]
        n208 = Index Array(array=w457, index=w452) -> (element=w454:string)
        n209 = Concatenate Strings(w454, "\r\n" ("write buffer")) -> (w453:string)
        n210 = Increment(x=w452) -> (x+1=w451:u8)
        n211 = Enqueue Element(queue=w456, element=w453) -> ()  [unwired: 2 in, 3 out]
        n212 = property on="Line" class="Slide (strict)"("Val(Sgnl)"=w451) -> ()  [unwired: 2 in, 2 out]
      }
      event "Grab Script": Value Change {
        w459 = u8 0 ("Line")
        n213 = event-data() -> ()  [unwired: 1 in, 1 out]
        n214 = property on="Line" class="Slide (strict)"("Val(Sgnl)"=w459) -> ()  [unwired: 2 in, 2 out]
        n215 = local read "Script"() -> (w460:string)
        n216 = property on="Notepad" class="Str"("Value"=w460, "Text.Scroll Position"=w459) -> ()  [unwired: 2 in, 2 out]
      }
      event Key Down {
        n217 = event-data() -> ("Char"=w470:i16, "VKey"=w469:T10, "ScanCode"=w468:i16, "Mods"=w467:cluster{"Num Pad":bool, "Menu Key":bool}, "PlatMods"=w466:T11, "FocusObj"=w463:refnum<vi>)  [unwired: 1 in]
        n218 = control-ref of="Console"() -> (w461:refnum<vi>)
        n219 = Bundle("Char"=w470, "VKey"=w469, "ScanCode"=w468, "Mods"=w467, "PlatMods"=w466, "FocusObj"=w463) -> (w462:T12)  [unwired: 1 in]
        n220 = Equal?(x=w463, y=w461) -> (x = y?=w465:bool)
        n221 = case shown="True" w465 {
          tunnel: w462 -> [_ w475]
          tunnel: w464 -> [_ w473]
          frame False {
          }
          frame True {
            n222 = call "TranslateTyping.vi"("Cluster"=w475) -> ("Extras"=w471:enum16{"Nix", "clear"}, "string"=w474:string)  [unwired: 9 in]
            n223 = case shown="\"Nix\", Default" w471 {
              tunnel: w473 -> [w476 w479]
              tunnel: [w476 w478] -> w472
              frame "Nix", Default {
              }
              frame "clear" {
                n224 = Enqueue Element(queue=w479, element="cline") -> (queue out=w478:refnum<queue>)  [unwired: 2 in, 2 out]
              }
            }
            n225 = Enqueue Element(queue=w472, element=w474) -> ()  [unwired: 2 in, 3 out]
          }
        }
      }
    }
  }
  n226 = property on="a" class="WFGraph (strict)"("Active Cursor"=u32 0, "Cursor.Cursor X"=-40.0 ("Cursor.Cursor Position:Cursor X"), "Active Cursor"=u32 1, "Cursor.Cursor X"=40.0 ("Cursor.Cursor Position:Cursor X")) -> ()  [unwired: 2 in, 2 out]
  n227 = property on="b" class="WFGraph (strict)"("Active Cursor"=u32 0, "Cursor.Cursor X"=-40.0 ("Cursor.Cursor Position:Cursor X"), "Active Cursor"=u32 1, "Cursor.Cursor X"=40.0 ("Cursor.Cursor Position:Cursor X")) -> ()  [unwired: 2 in, 2 out]
